vi "test-path-planner-read-csv.vi"() -> ()   [LabVIEW 2019]
uses:
  <vilib>/Rock Robotics/WPI/ThirdParty/MJansen/PathPlanner/PathPlannerTrajectory.ctl
  <vilib>/Rock Robotics/WPI/ThirdParty/MJansen/PathPlanner/PathPlannerState.ctl
  <vilib>/Rock Robotics/WPI/ThirdParty/JAS_Junk/TrajLib/TypeDef/ROTATION2D.ctl
  <vilib>/Rock Robotics/WPI/ThirdParty/JAS_Junk/TrajLib/TypeDef/TRAJ_STATE.ctl
  <vilib>/Rock Robotics/WPI/ThirdParty/JAS_Junk/TrajLib/TypeDef/POSE2D.ctl
  <vilib>/Rock Robotics/WPI/ThirdParty/JAS_Junk/TrajLib/TypeDef/TRANSLATION2D.ctl
  <vilib>/Rock Robotics/WPI/ThirdParty/MJansen/PathPlanner/PathPlanner.lvlib
  <vilib>/Rock Robotics/WPI/ThirdParty/JAS_Junk/TrajLib/Trajectory_Library.lvlib
panel:
  in  "Tab Control":T1(tab)
  in  "stop":bool
  in  "Path FileName":string="C:\\Shares\\github\\PathPlannerLabVIEW\\PathPlannerSandbox\\PathPlannerTestCSV\\PathPlannerTestCSV.csv"
  out "Full FIlename":string
  out "error out":errorcluster
  out "PathPlannerTrajectory":T2 {"States"."HolonomicAngular\nvelocity Deg/Sec"."SIN" format="%13.4f"; "States"."HolonomicAngular\nvelocity Deg/Sec"."COS" format="%13.4f"; "States"."HolonomicAngular\nvelocity Deg/Sec"."VALUE" format="%13.4f"; "States"."HolonomicRotation"."SIN" format="%13.4f"; "States"."HolonomicRotation"."COS" format="%13.4f"; "States"."HolonomicRotation"."VALUE" format="%13.4f"; "States"."AngularVelocity"."SIN" format="%13.4f"; "States"."AngularVelocity"."COS" format="%13.4f"; "States"."AngularVelocity"."VALUE" format="%13.4f"; "States"."TrajectoryState"."POSE"."ROTATION"."SIN" format="%13.4f"; "States"."TrajectoryState"."POSE"."ROTATION"."COS" format="%13.4f"; "States"."TrajectoryState"."POSE"."ROTATION"."VALUE" format="%13.4f"; "States"."TrajectoryState"."POSE"."TRANSLATION"."Y" format="%14.3f"; "States"."TrajectoryState"."POSE"."TRANSLATION"."X" format="%14.3f"; "States"."AngularAcceleration"."SIN" format="%13.4f"; "States"."AngularAcceleration"."COS" format="%13.4f"; "States"."AngularAcceleration"."VALUE" format="%13.4f"}
  out "outPathPlannerStates":T3[](array[typedef]) {"HolonomicAngular\nvelocity Deg/Sec"."SIN" format="%13.4f"; "HolonomicAngular\nvelocity Deg/Sec"."COS" format="%13.4f"; "HolonomicAngular\nvelocity Deg/Sec"."VALUE" format="%13.4f"; "HolonomicRotation"."SIN" format="%13.4f"; "HolonomicRotation"."COS" format="%13.4f"; "HolonomicRotation"."VALUE" format="%13.4f"; "AngularVelocity"."SIN" format="%13.4f"; "AngularVelocity"."COS" format="%13.4f"; "AngularVelocity"."VALUE" format="%13.4f"; "TrajectoryState"."POSE"."ROTATION"."SIN" format="%13.4f"; "TrajectoryState"."POSE"."ROTATION"."COS" format="%13.4f"; "TrajectoryState"."POSE"."ROTATION"."VALUE" format="%13.4f"; "TrajectoryState"."POSE"."TRANSLATION"."Y" format="%14.3f"; "TrajectoryState"."POSE"."TRANSLATION"."X" format="%14.3f"; "AngularAcceleration"."SIN" format="%13.4f"; "AngularAcceleration"."COS" format="%13.4f"; "AngularAcceleration"."VALUE" format="%13.4f"}
  in  "Down Button":bool
  in  "Up Button":bool
  in  "index":i32 step=20
  out "LabVIEWStateCount":i32
  out "LabVIEWStates":T5[](array[typedef]) {"POSE"."ROTATION"."SIN" format="%13.4f"; "POSE"."ROTATION"."COS" format="%13.4f"; "POSE"."ROTATION"."VALUE" format="%13.4f"; "POSE"."TRANSLATION"."Y" format="%14.3f"; "POSE"."TRANSLATION"."X" format="%14.3f"}
  out "XY SPLINE":cluster{dbl[], dbl[]}[](graph)
  out "XY Graph":cluster{dbl[], dbl[]}[](graph)
  out "Sample Graph":dbl[][](graph)
  out "LabVIEW Time Plot":cluster{dbl[], dbl[]}[](graph)
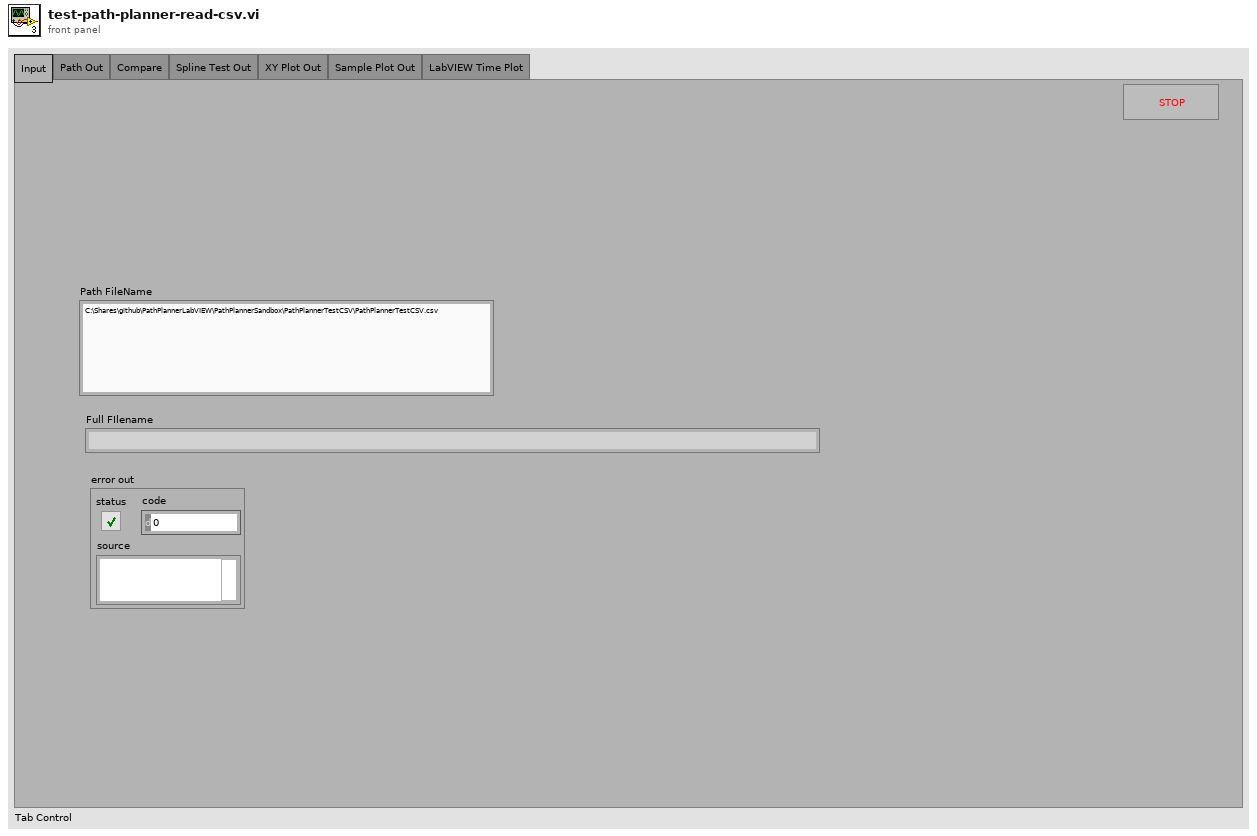
[diagram p1: front panel]
types:
  T1 = enum32{"Input", "Path Out", "Compare", "Spline Test Out", "XY Plot Out", "Sample Plot Out", "LabVIEW Time Plot"}
  T2 = typedef "PathPlanner.lvlib/PathPlannerTrajectory.ctl" = cluster{"TotalTimeSeconds":dbl, "States":T3[]}
  T3 = typedef "PathPlanner.lvlib/PathPlannerState.ctl" = cluster{"AngularAcceleration":T4, "PositionMeters":dbl, "TrajectoryState":T5, "AngularVelocity":T4, "HolonomicRotation":T4, "CurveRadius":dbl, "DeltaPos":dbl, "HolonomicAngular\nvelocity Deg/Sec":T4}
  T4 = typedef "Trajectory_Library.lvlib/ROTATION2D.ctl" = cluster{"VALUE":dbl, "COS":dbl, "SIN":dbl}
  T5 = typedef "Trajectory_Library.lvlib/TRAJ_STATE.ctl" = cluster{"TimeSeconds":dbl, "Velocity":dbl, "Acceleration":dbl, "POSE":T6, "Curvature":dbl}
  T6 = typedef "Trajectory_Library.lvlib/POSE2D.ctl" = cluster{"TRANSLATION":T7, "ROTATION":T4}
  T7 = typedef "Trajectory_Library.lvlib/TRANSLATION2D.ctl" = cluster{"X":dbl, "Y":dbl}
  T8 = typedef "Trajectory_Library.lvlib/TRAJECTORY.ctl" = cluster{"TotalTImeSecs":dbl, "States":T5[]}
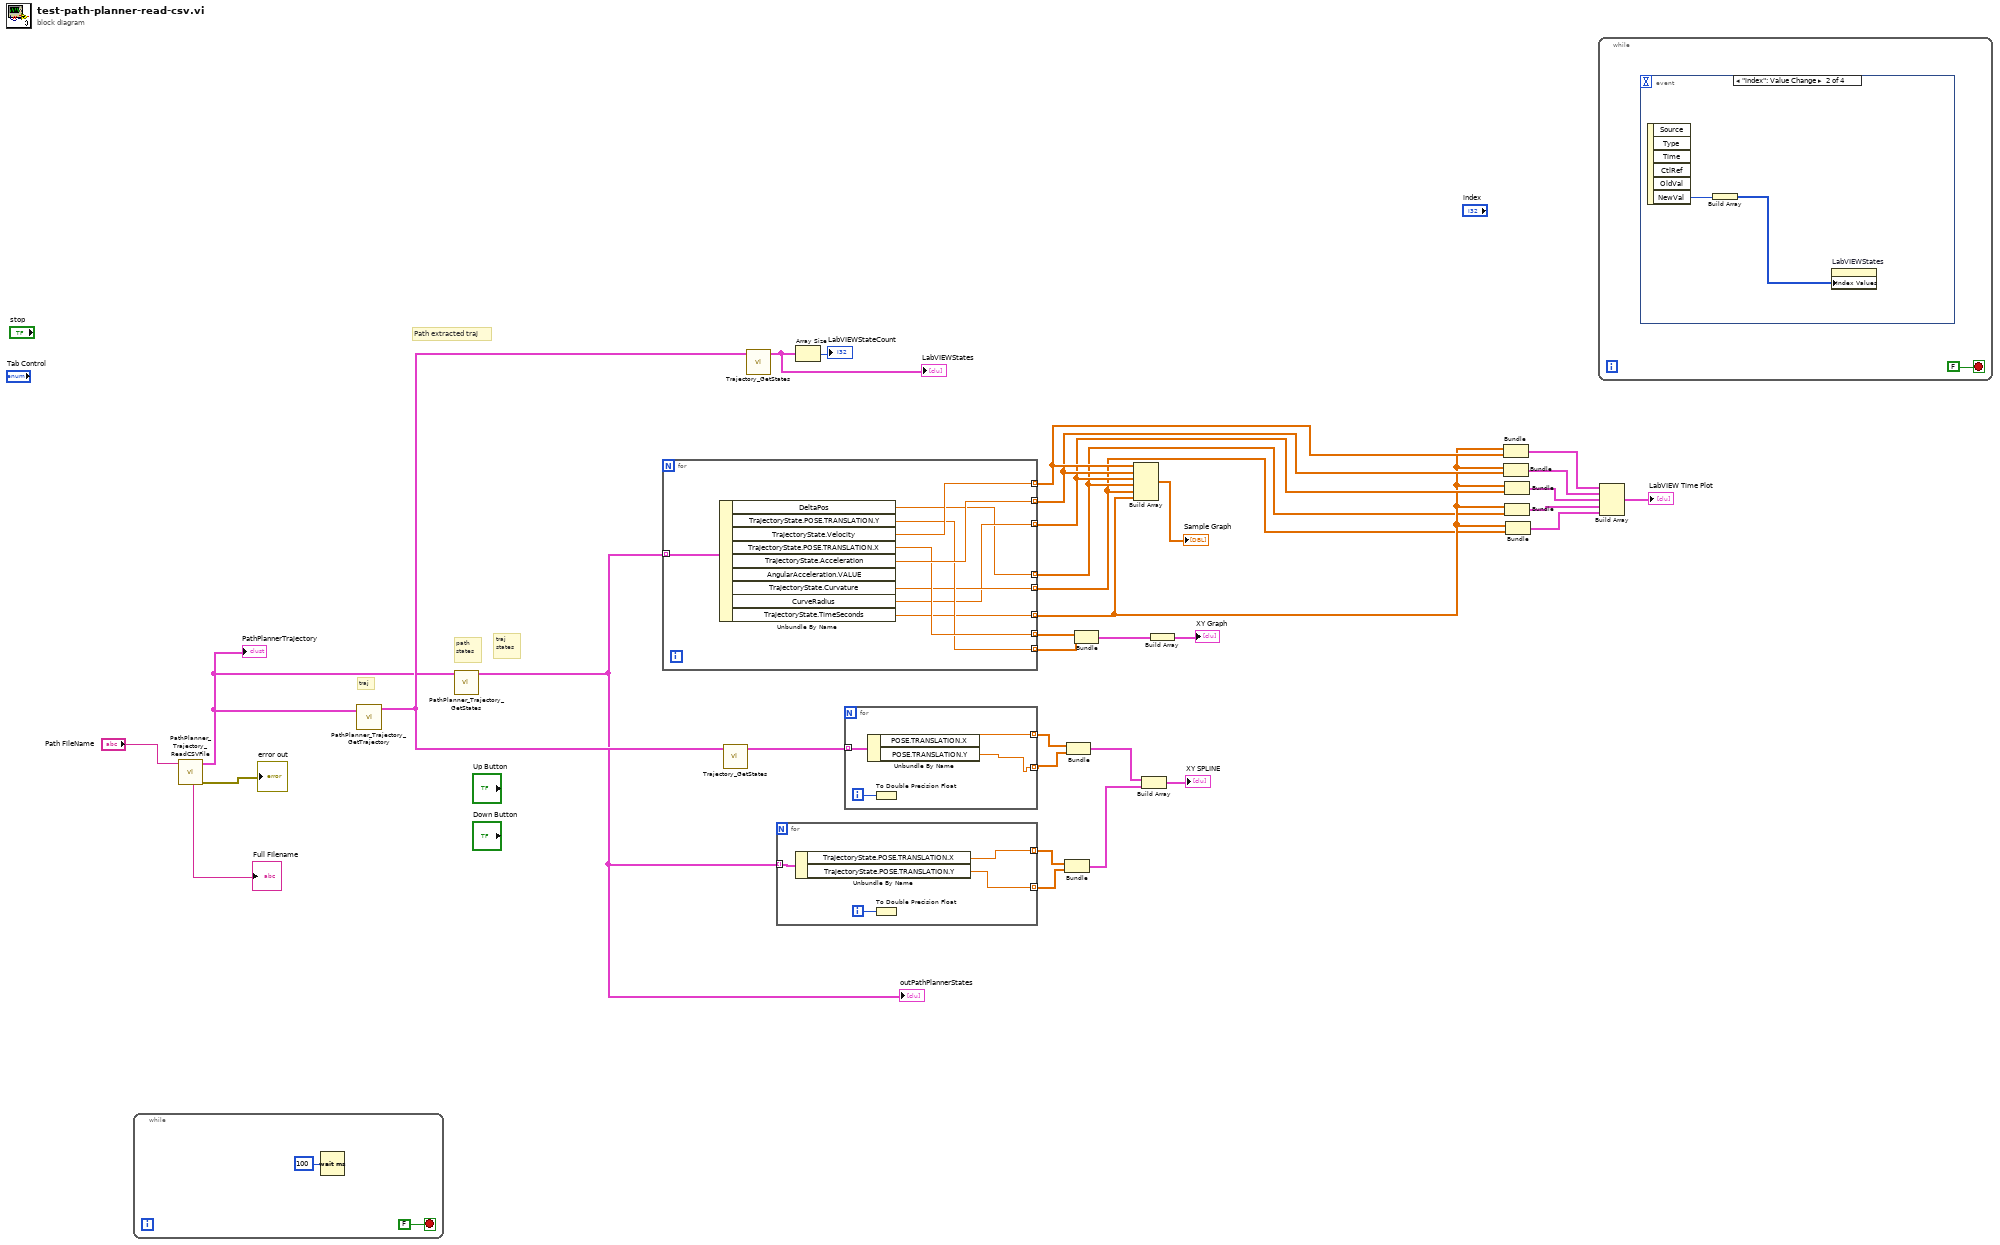
[diagram p0: block diagram]
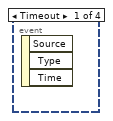
[diagram p2: hidden frame]
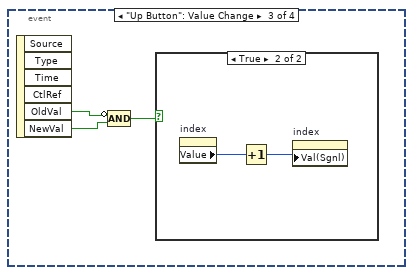
[diagram p3: hidden frame]
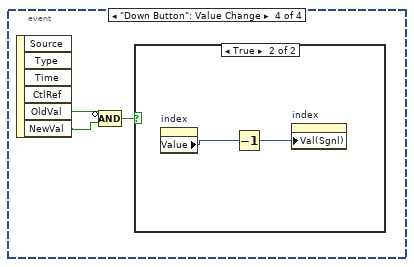
[diagram p5: hidden frame]
diagram:
  # "Path extracted traj"
  # "traj"
  # "traj\nstates"
  # "path\nstates"
  n1 = while {
    stop <- FALSE stop-if-true
    n2 = Wait (ms)(milliseconds to wait=u32 100) -> ()  [unwired: 1 out]
  }
  n3 = call <vilib>:"PathPlanner_Trajectory_ReadCSVFile.vi"("FileName"="Path FileName") -> ("error out"=→"error out":errorcluster, "outTRAJECTORY"=w3:T2, "Full FIlename"=→"Full FIlename":string)  [unwired: 8 in]
  "PathPlannerTrajectory" <- w3
  n4 = call <vilib>:"PathPlanner_Trajectory_GetTrajectory.vi"("PathPlannerTrajectory"=w3) -> ("TRAJECTORY"=w20:T8)  [unwired: 10 in]
  n5 = call <vilib>:"PathPlanner_Trajectory_GetStates.vi"("PathPlannerTrajectory"=w3) -> ("PathPlannerStates"=w17:T3[])  [unwired: 10 in]
  "outPathPlannerStates" <- w17
  n6 = for {
    tunnel: [w44] -> w15 mode=indexing
    tunnel: [w43] -> w14 mode=indexing
    tunnel: [w37] -> w11 mode=indexing
    tunnel: [w42] -> w32 mode=indexing
    tunnel: [w41] -> w31 mode=indexing
    tunnel: w17 -> [w40] mode=indexing
    tunnel: [w39] -> w10 mode=indexing
    tunnel: [w38] -> w13 mode=indexing
    tunnel: [w36] -> w12 mode=indexing
    n7 = Unbundle By Name(w40) -> ("DeltaPos"=w37:dbl, "TrajectoryState.POSE.TRANSLATION.Y"=w41:dbl, "TrajectoryState.Velocity"=w44:dbl, "TrajectoryState.POSE.TRANSLATION.X"=w42:dbl, "TrajectoryState.Acceleration"=w43:dbl, "TrajectoryState.Curvature"=w39:dbl, "CurveRadius"=w38:dbl, "TrajectoryState.TimeSeconds"=w36:dbl)  [unwired: 1 out]
  }
  n8 = call <vilib>:"Trajectory_GetStates.vi"("TRAJECTORY"=w20) -> ("States"=w21:T5[])  [unwired: 10 in]
  n9 = call <vilib>:"Trajectory_GetStates.vi"("TRAJECTORY"=w20) -> ("States"=w18:T5[])  [unwired: 10 in]
  "LabVIEWStates" <- w18
  n10 = for {
    tunnel: [w47] -> w26 mode=indexing
    tunnel: w17 -> [w46] mode=indexing
    tunnel: [w45] -> w25 mode=indexing
    i -> [w48]
    n11 = Unbundle By Name(w46) -> ("TrajectoryState.POSE.TRANSLATION.X"=w47:dbl, "TrajectoryState.POSE.TRANSLATION.Y"=w45:dbl)
    n12 = To Double Precision Float(number=w48) -> ()  [unwired: 1 out]
  }
  n13 = Array Size(array=w18) -> (size(s)=→"LabVIEWStateCount":i32)
  n14 = for {
    tunnel: [w51] -> w28 mode=indexing
    tunnel: [w50] -> w27 mode=indexing
    tunnel: w21 -> [w49] mode=indexing
    i -> [w52]
    n15 = Unbundle By Name(w49) -> ("POSE.TRANSLATION.X"=w51:dbl, "POSE.TRANSLATION.Y"=w50:dbl)
    n16 = To Double Precision Float(number=w52) -> ()  [unwired: 1 out]
  }
  n17 = Bundle(w26, w25) -> (w23:cluster{dbl[], dbl[]})  [unwired: 1 in]
  n18 = Bundle(w28, w27) -> (w24:cluster{dbl[], dbl[]})  [unwired: 1 in]
  n19 = Bundle(w32, w31) -> (w30:cluster{dbl[], dbl[]})  [unwired: 1 in]
  n20 = Build Array(w15, w14, w13, w11, w10, w12) -> (→"Sample Graph":dbl[][])
  n21 = Build Array(w24, w23) -> (→"XY SPLINE":cluster{dbl[], dbl[]}[])
  n22 = Build Array(w30) -> (→"XY Graph":cluster{dbl[], dbl[]}[])
  n23 = Bundle(w12, w15) -> (w9:cluster{dbl[], dbl[]})  [unwired: 1 in]
  n24 = Bundle(w12, w14) -> (w8:cluster{dbl[], dbl[]})  [unwired: 1 in]
  n25 = Bundle(w12, w13) -> (w7:cluster{dbl[], dbl[]})  [unwired: 1 in]
  n26 = Bundle(w12, w11) -> (w6:cluster{dbl[], dbl[]})  [unwired: 1 in]
  n27 = Bundle(w12, w10) -> (w5:cluster{dbl[], dbl[]})  [unwired: 1 in]
  n28 = while {
    stop <- FALSE stop-if-true
    n29 = event shown="[1] \"index\": Value Change" {
      selector: _ -> [_ _ _ _]
      dyn-events: _ -> [_ _ _ _]
      timeout: _ -> [_ _ _ _]
      event Timeout {
        n30 = event-data() -> ()  [unwired: 1 in, 3 out]
      }
      event "index": Value Change {
        n31 = event-data() -> ("NewVal"=w55:i32)  [unwired: 1 in, 5 out]
        n32 = Build Array(w55) -> (w54:i32[])
        n33 = property on="LabVIEWStates" class="Arr (strict)"("Index Values"=w54) -> ()  [unwired: 2 in, 2 out]
      }
      event "Up Button": Value Change {
        n34 = event-data() -> ("OldVal"=w58:bool, "NewVal"=w57:bool)  [unwired: 1 in, 4 out]
        n35 = Compound Arithmetic op=AND(invert w58, w57) -> (w56:bool)
        n36 = case shown="True" w56 {
          frame False {
          }
          frame True {
            n37 = property on="index" class="DigNum (strict)"() -> ("Value"=w59:i32)  [unwired: 2 in, 2 out]
            n38 = Increment(x=w59) -> (x+1=w60:i32)
            n39 = property on="index" class="DigNum (strict)"("Val(Sgnl)"=w60) -> ()  [unwired: 2 in, 2 out]
          }
        }
      }
      event "Down Button": Value Change {
        n40 = event-data() -> ("OldVal"=w62:bool, "NewVal"=w61:bool)  [unwired: 1 in, 4 out]
        n41 = Compound Arithmetic op=AND(invert w62, w61) -> (w63:bool)
        n42 = case shown="True" w63 {
          frame False {
          }
          frame True {
            n43 = property on="index" class="DigNum (strict)"() -> ("Value"=w64:i32)  [unwired: 2 in, 2 out]
            n44 = Decrement(x=w64) -> (x-1=w65:i32)
            n45 = property on="index" class="DigNum (strict)"("Val(Sgnl)"=w65) -> ()  [unwired: 2 in, 2 out]
          }
        }
      }
    }
  }
  n46 = Build Array(w9, w8, w7, w6, w5) -> (→"LabVIEW Time Plot":cluster{dbl[], dbl[]}[])
